vi "tokens to path.vi"(10 "Data Access:OS":T1, 11 "array of strings":string[](array[string])) -> (3 "String":string)   [LabVIEW 2013, in "PL Framework Configuration Tool.lvlib"]
uses:
  PL Framework Configuration Tool.lvlib
  <vilib>/NI/Tag Bus Module Framework/root configuration/Target Types.ctl
  <vilib>/NI/Tag Bus Module Framework/root configuration/TBM configuration.lvclass
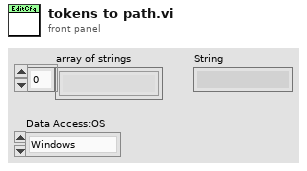
[diagram p1: front panel]
types:
  T1 = typedef "TBM configuration.lvclass/Target Types.ctl" = enum16{"Windows", "Mac", "Linux", "Linux RT ARM", "VxWorks", "Pharlap", "Other", "Linux RT x64"}
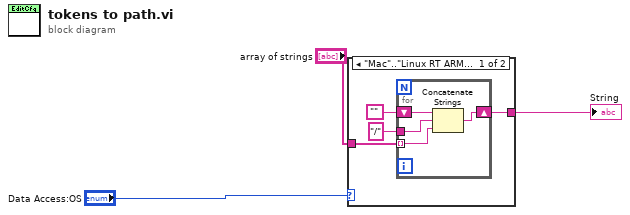
[diagram p0: block diagram]
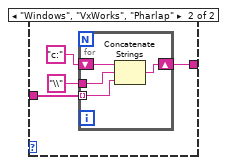
[diagram p2: hidden frame]
diagram:
  n1 = case shown="\"Mac\"..\"Linux RT ARM\", \"Other\", \"Linux RT x64\"" "Data Access:OS" {
    tunnel: "array of strings" -> [w7 w14]
    tunnel: [w6 w13] -> w3
    frame "Mac".."Linux RT ARM", "Other", "Linux RT x64" {
      n2 = for {
        tunnel: w7 -> [w10] mode=indexing
        shift-right: [w9] -> w6
        shift-left: "" -> [w11]
        tunnel: "/" -> [w8]
        n3 = Concatenate Strings(w11, w8, w10) -> (w9:string)
      }
    }
    frame "Windows", "VxWorks", "Pharlap" {
      n4 = for {
        tunnel: w14 -> [w18] mode=indexing
        shift-right: [w17] -> w13
        shift-left: "c:" -> [w19]
        tunnel: "\\" -> [w16]
        n5 = Concatenate Strings(w19, w16, w18) -> (w17:string)
      }
    }
  }
  "String" <- w3
